vi "Get Source Path From Install Path.vi"(8 "Error In":errorcluster, 10 "Install File Path":path, 11 "Configuration":T1) -> (0 "Error Out":errorcluster, 1 "Source File Path":path, 2 "Install File Path":path, 3 "Configuraiton":T1)   [LabVIEW 2011, in "LVH-Build-Tools.lvlib"]
doc: "Get the source path of a file based on its install path.\n\nThis VI strips the install root path from the file path and prepends the source path."
uses:
  LVH-Build-Tools.lvlib
  Type Defs/Configuration.ctl
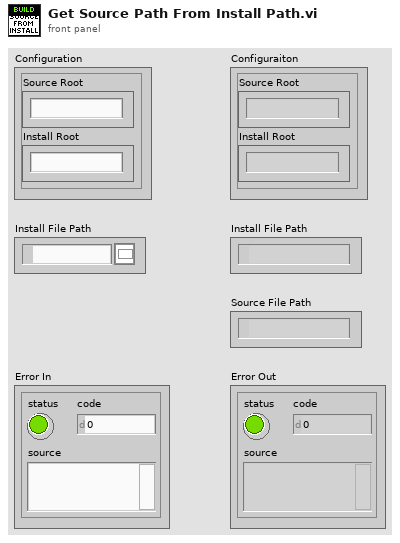
[diagram p1: front panel]
types:
  T1 = typedef "LVH-Build-Tools.lvlib/Configuration.ctl" = cluster{"Source Root":string, "Install Root":string, "Components":string[], "Ignore":string[]}
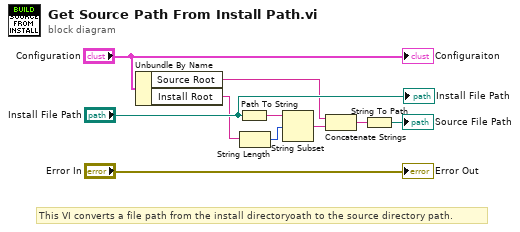
[diagram p0: block diagram]
diagram:
  # "This VI converts a file path from the install directoryoath to the source directory path."
  n1 = Unbundle By Name("Configuration") -> ("Source Root"=w3:string, "Install Root"=w2:string)
  n2 = Path To String(path="Install File Path") -> (string=w8:string)
  n3 = String Length(string=w2) -> (length=w9:i32)
  n4 = String Subset(string=w8, offset (0)=w9) -> (substring=w10:string)  [unwired: 1 in]
  n5 = Concatenate Strings(w3, w10) -> (w5:string)
  n6 = String To Path(string=w5) -> (path=→"Source File Path":path)
  "Error Out" <- "Error In"
  "Configuraiton" <- "Configuration"
  "Install File Path" <- "Install File Path"
